vi "Set ni_xnet_can_bm_api_StopProcessReply.vi"(7 "Complete Call (T)":bool=TRUE, 8 "error in (no error)":errorcluster, 10 "package_templatemessage":T1, 11 "gRPCid":T3) -> (0 "error out":errorcluster)   [LabVIEW 2025, in "xnet_can_bus_monitor_api_server.lvlib"]
uses:
  xnet_can_bus_monitor_api_server.lvlib
  <vilib>/gRPC/LabVIEW gRPC Library/Shared/grpcId.ctl
  ni_xnet_can_bm_api_StopProcessReply.ctl
  ni_xnet_can_bm_api_ErrorInfo.ctl
  ni_xnet_can_bm_api_StopProcessReply_Flat.ctl
  ni_xnet_can_bm_api_ErrorInfo_Flat.ctl
  dcc74a39-081a-4bdd-860b-8ed792803c96.vi
  RichToFlatni_xnet_can_bm_api_ErrorInfo.vi
  <vilib>/gRPC/LabVIEW gRPC Library/Shared/TranslateGrpcError.vi
  <vilib>/gRPC/LabVIEW gRPC Library/Server API/Server/Get Server DLL Path.vi
  <vilib>/Utility/error.llb/Error Cluster From Error Code.vi
  <vilib>/gRPC/LabVIEW gRPC Library/grpc-lvsupport-release.lvlib
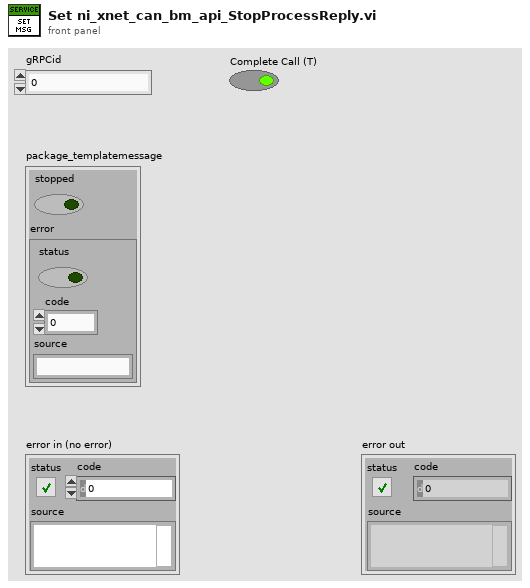
[diagram p1: front panel]
types:
  T1 = typedef "xnet_can_bus_monitor_api_server.lvlib/ni_xnet_can_bm_api_StopProcessReply.ctl" = cluster{"stopped":bool, "error":T2}
  T2 = typedef "xnet_can_bus_monitor_api_server.lvlib/ni_xnet_can_bm_api_ErrorInfo.ctl" = errorcluster
  T3 = typedef "grpc-lvsupport-release.lvlib/grpcId.ctl" = u64
  T4 = typedef "xnet_can_bus_monitor_api_server.lvlib/ni_xnet_can_bm_api_StopProcessReply_Flat.ctl" = cluster{"stopped":bool, "error":T5}
  T5 = typedef "xnet_can_bus_monitor_api_server.lvlib/ni_xnet_can_bm_api_ErrorInfo_Flat.ctl" = errorcluster
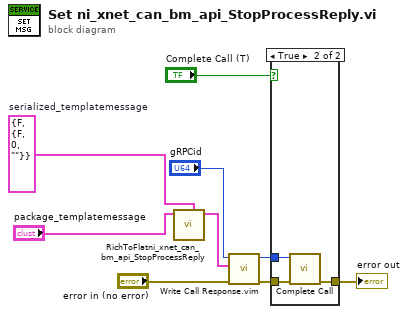
[diagram p0: block diagram]
diagram:
  w2 = T4 {"stopped"=FALSE, "error"={"status"=FALSE, "code"=0, "source"=""}}  # serialized_templatemessage
  n1 = call "RichToFlatni_xnet_can_bm_api_StopProcessReply.vi"("OutputClusterType"=w2, "InputCluster"="package_templatemessage") -> ("OutputCluster"=w1:T4)  [unwired: 9 in]
  n2 = call "Write Call Response.vim"("error in"="error in (no error)", "Response Data"=w1, "gRPCid in"="gRPCid") -> ("error out"=w6:errorcluster, "gRPCid out"=w7:T3)  [unwired: 7 in]
  n3 = case shown="True" "Complete Call (T)" {
    tunnel: [w10 w13] -> w9
    tunnel: w7 -> [_ w12]
    tunnel: w6 -> [w10 w11]
    frame False {
    }
    frame True {
      n4 = call <vilib>:"Complete Call.vi"("gRPCid"=w12, "error in"=w11) -> ("error out"=w13:errorcluster)  [unwired: 8 in]
    }
  }
  "error out" <- w9
